vi "Write Running Internal Data.vi"(8 "error in (no error)":errorcluster, 10 "Running Internal Data":T1={"Refresh"=TRUE, "Iterations"=0, "Housekeep only"=FALSE, "Configured period (ns)"=0}, 11 "CIFCorePlugin in":refnum<class "CIFCorePlugin.lvclass">) -> (0 "error out":errorcluster, 3 "CIFCorePlugin out":refnum<class "CIFCorePlugin.lvclass">)   [LabVIEW 2021, in "CIFCorePlugin.lvclass"]
uses:
  CIFCorePlugin.lvclass
  Typedef/Running Internal Data.ctl
  CIFCorePlugin.lvclass/CIFCorePlugin.ctl
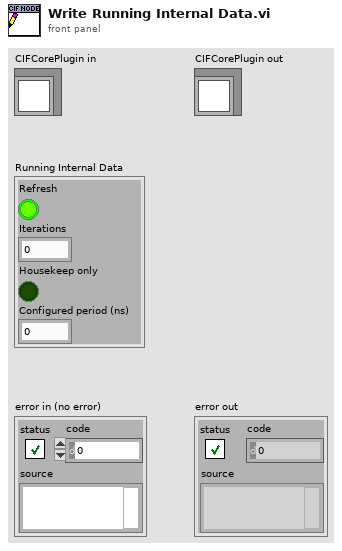
[diagram p1: front panel]
types:
  T1 = typedef "CIFCorePlugin.lvclass/Running Internal Data.ctl" = cluster{"Refresh":bool, "Iterations":i64, "Housekeep only":bool, "Configured period (ns)":i64}
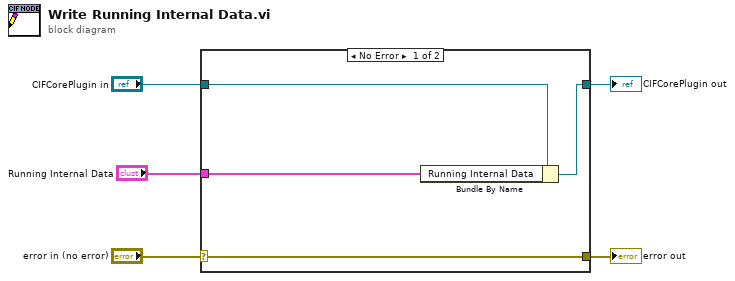
[diagram p0: block diagram]
diagram:
  n1 = case shown="No Error" "error in (no error)" {
    selector: "error in (no error)" -> [w9 w10]
    tunnel: [w9 w10] -> w4
    tunnel: [w7 w11] -> w2
    tunnel: "CIFCorePlugin in" -> [w8 w11]
    tunnel: "Running Internal Data" -> [w6 _]
    frame No Error {
      n2 = Bundle By Name(cluster=w8, "Running Internal Data"=w6) -> (w7:refnum<class "CIFCorePlugin.lvclass">)
    }
    frame Error {
    }
  }
  "error out" <- w4
  "CIFCorePlugin out" <- w2
